vi "MAT Save Matrix Header.vi"(4 "Real/Complex (0-Real)":u32, 6 "Rep. Code":u32, 7 "offset in (-1: current position)":i64=-1, 8 "error in (no error)":errorcluster, 9 "Matrix Size":i32[](array[numeric]), 10 "Matrix Name":string, 11 "Ref Num":refnum<file>) -> (0 "error out":errorcluster, 2 "offset out":i64, 3 "Dup Ref Num":refnum<file>)   [LabVIEW 2018]
doc: "Matlab mat-v4 lib: Writes header for variable of given type and name to file. If the 'offset in' is assigned it will set file position to the offset. If the value is -1 (default) it will write to current position. 'offset out' is byte offset after the header where data should be written."
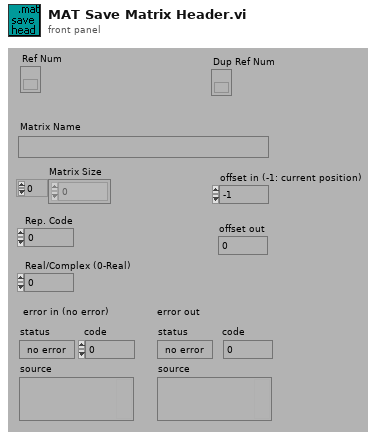
[diagram p1: front panel]
types:
  T1 = enum16{"big-endian, network order", "native, host order", "little-endian"}
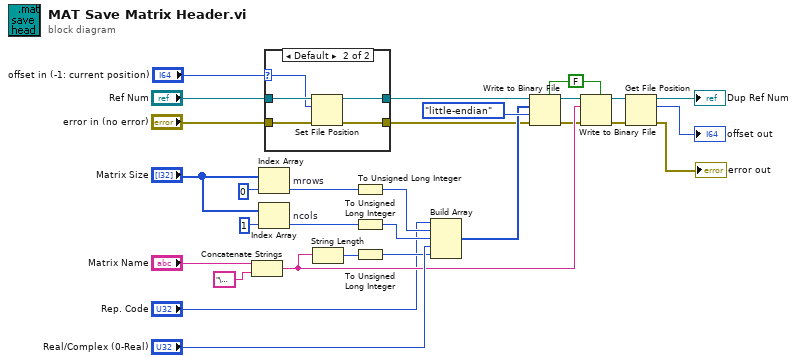
[diagram p0: block diagram]
diagram:
  w7 = FALSE ("prepend array or string size? (T)")
  n1 = Concatenate Strings("Matrix Name", "\u0000") -> (w17:string)
  n2 = Index Array "mrows"(array="Matrix Size", index=0) -> (element=w25:i32)
  n3 = Index Array "ncols"(array="Matrix Size", index=1) -> (element=w26:i32)
  n4 = case shown="Default" "offset in (-1: current position)" {
    selector: "offset in (-1: current position)" -> [_ w32]
    tunnel: "error in (no error)" -> [w30 w36]
    tunnel: [w30 w35] -> w5
    tunnel: [w31 w34] -> w4
    tunnel: "Ref Num" -> [w31 w33]
    frame -1 {
    }
    frame Default {
      n5 = Set File Position(offset (in bytes) (0)=w32, refnum=w33, error in=w36) -> (refnum out=w34:refnum<file>, error out=w35:errorcluster)  [unwired: 1 in]
    }
  }
  n6 = String Length(string=w17) -> (length=w18:i32)
  n7 = To Unsigned Long Integer(number=w25) -> (unsigned 32bit integer=w24:u32)
  n8 = To Unsigned Long Integer(number=w26) -> (unsigned 32bit integer=w23:u32)
  n9 = To Unsigned Long Integer(number=w18) -> (unsigned 32bit integer=w21:u32)
  n10 = Build Array("Rep. Code", w24, w23, "Real/Complex (0-Real)", w21) -> (w10:u32[])
  n11 = Write to Binary File(file (use dialog)=w4, data=w10, error in=w5, 5:w7, 9:T1."little-endian" ("byte order (0:big-endian, network order)")) -> (refnum out=w8:refnum<file>, error out=w9:errorcluster)  [unwired: 1 in, 1 out]
  n12 = Write to Binary File(file (use dialog)=w8, data=w17, error in=w9, 5:w7) -> (refnum out=w13:refnum<file>, error out=w12:errorcluster)  [unwired: 2 in, 1 out]
  n13 = Get File Position(4:w12, 7:w13) -> (0:→"error out":errorcluster, 2:→"offset out":i64, 3:→"Dup Ref Num":refnum<file>)
